vi "Test Create Formatter.vi"(8 "error in":errorcluster) -> (0 "error out":errorcluster)   [LabVIEW 2016, in "UT_Formatter.lvlib"]
doc: "Test creation of the default formatter."
uses:
  UT_Formatter.lvlib
  Source/HSE-Logger/LogLevel.ctl
  Source/HSE-Logger/Handler/FileHandler/FileHandler.lvclass/FileHandler.ctl
  Source/HSE-Logger/Handler/FileHandler/FileHandler.lvclass
  <vilib>/addons/_JKI Toolkits/Caraya/classes/Test/Test.lvclass
  Source/HSE-Logger/hse-logger.lvlib
  Source/HSE-Logger/Formatter/Formatter.lvclass
  <vilib>/addons/_JKI Toolkits/Caraya/classes/Assert/Assert.lvclass
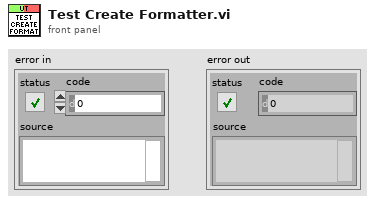
[diagram p1: front panel]
types:
  T1 = typedef "hse-logger.lvlib/LogLevel.ctl" = enum16{"DEBUG", "INFO", "WARNING", "ERROR", "CRITICAL"}
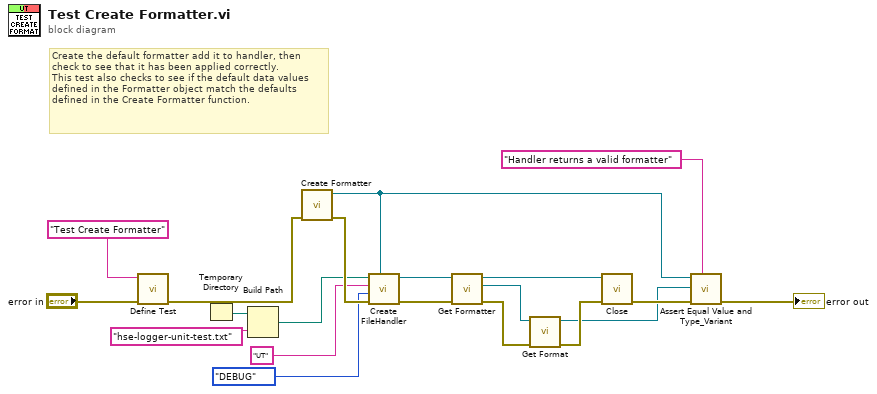
[diagram p0: block diagram]
diagram:
  # "Create the default formatter add it to handler, then check to see that it has been applied correctly.\nThis test also checks to see if the default data values defined in the Formatter object match the defaults defined in the Create Formatter function."
  n1 = call <vilib>:"Define Test.vi"("error in (no error)"="error in", "Label (VI Title)"="Test Create Formatter") -> ("error out"=w16:errorcluster)  [unwired: 8 in, 1 out]
  n2 = Temporary Directory() -> (w4:path)
  n3 = Build Path(base path=w4, name or relative path="hse-logger-unit-test.txt") -> (appended path=w3:path)
  n4 = call "Create Formatter.vi"("error in"=w16) -> ("error out"=w13:errorcluster, "Formatter out"=w5:refnum<class "Formatter.lvclass">)  [unwired: 9 in]
  n5 = call "Create FileHandler.vi"("Formatter.lvclass"=w5, "error in"=w13, "Level"=LogLevel."DEBUG", "Name"="UT", "Filepath"=w3) -> ("error out"=w9:errorcluster, "FileHandler out"=w10:refnum<class "FileHandler.lvclass">)  [unwired: 5 in]
  n6 = call "Get Formatter.vi"("error in"=w9, "FileHandler"=w10) -> ("error out"=w7:errorcluster, "Formatter"=w6:refnum<class "Formatter.lvclass">, "FileHandler out"=w8:refnum<class "FileHandler.lvclass">)  [unwired: 7 in]
  n7 = call "Get Format.vi"("error in"=w7, "Formatter in"=w6) -> ("error out"=w19:errorcluster, "Formatter out"=w1:refnum<class "Formatter.lvclass">)  [unwired: 7 in, 1 out]
  n8 = call-dynamic "Close.vi"("error in"=w19, "FileHandler in"=w8) -> ("error out"=w18:errorcluster)  [unwired: 8 in, 1 out]
  n9 = call <vilib>:"Assert Equal Value and Type_Variant.vi"("Label"="Handler returns a valid formatter", "error in (no error)"=w18, "Y"=w1, "X"=w5) -> ("error out"=→"error out":errorcluster)  [unwired: 6 in, 1 out]
